vi "Actor Queue.vi"(6 "Creator Queue":refnum<data-value>, 8 "Creator Queue Alias":string, 9 "Self Queue Alias":string, 10 "Queue of Self Queue":refnum<queue>, 11 "Queue":refnum<class "Queue.lvclass">) -> ()   [LabVIEW 2021, in "jettl.lvlib" / "Base Queue.lvlib" / "Base Queue.lvclass"]
uses:
  Base Queue.lvclass
  Queue/Queue.lvclass
  C:/git/jettl/jettl/jettl/jettl/jettl.lvclass
  Msg Strategy/Msg Strategy.lvclass
  C:/git/jettl/jettl/jettl/Queue/Queue.lvclass
  Base Queue.lvclass/Base Queue.ctl
  Self Queue/Self Queue.lvlib
  jettl.lvlib
  Queue Mailbox/Queue Mailbox.lvlib
  Last Ack Created Queue Msg Strategy/Last Ack Created Queue Msg Strategy.lvlib
  Last Ack Creator Queue Msg Strategy/Last Ack Creator Queue Msg Strategy.lvlib
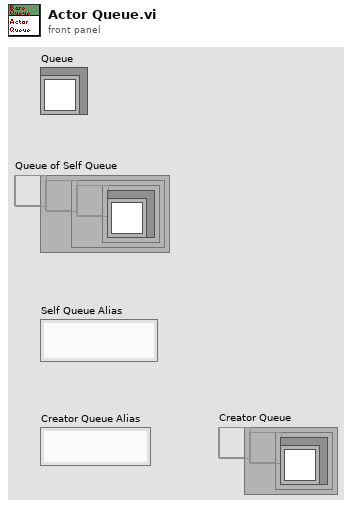
[diagram p1: front panel]
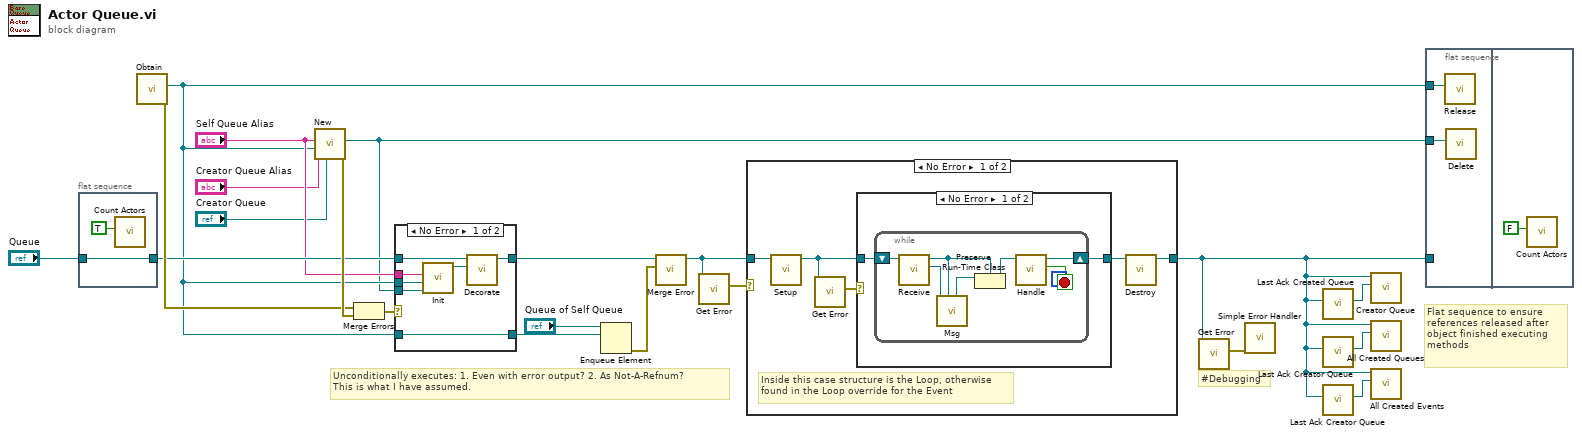
[diagram p0: block diagram]
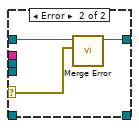
[diagram p2: hidden frame]
diagram:
  # "Flat sequence to ensure references released after object finished executing methods"
  # "#Debugging"
  # "Unconditionally executes: 1. Even with error output? 2. As Not-A-Refnum?\nThis is what I have assumed."
  n1 = flat-sequence {
    tunnel: [w22] -> w11
    tunnel: "Queue" -> [w22]
    frame #0 {
      n2 = call "Count Actors.vi"("Increment?"=TRUE) -> ()  [unwired: 11 in]
    }
  }
  n3 = call "Obtain.vi"() -> ("error out"=w12:errorcluster, "Self Queue"=w8:refnum<data-value>)  [unwired: 10 in]
  n4 = call "New.vi"("Creator Queue"="Creator Queue", "Creator Queue Alias"="Creator Queue Alias", "Self Queue"=w8, "Self Queue Alias"="Self Queue Alias") -> ("error out"=w13:errorcluster, "Queue Mailbox"=w5:refnum<data-value>)  [unwired: 6 in]
  n5 = Merge Errors(w12, w13) -> (w14:errorcluster)
  n6 = case shown="No Error" w14 {
    selector: w14 -> [_ w32]
    tunnel: [w29 w33] -> w19
    tunnel: w11 -> [w30 w31]
    tunnel: w8 -> [w28 _]
    tunnel: [w28 _] -> w18
    tunnel: w5 -> [w26 _]
    tunnel: "Self Queue Alias" -> [w25 _]
    tunnel: w8 -> [w24 _]
    frame No Error {
      n7 = call "Init.vi"("Queue Mailbox"=w26, "Self Queue"=w24, "Self Queue Alias"=w25) -> ("Base Queue out"=w27:refnum<class "Base Queue.lvclass">)  [unwired: 8 in]
      n8 = call-dynamic "Decorate.vi"("Queue"=w27, "Queue in"=w30) -> ("Queue out"=w29:refnum<class "Queue.lvclass">)  [unwired: 9 in]
    }
    frame Error {
      n9 = call-dynamic "Merge Error.vi"("Error"=w32, "Merge Error in"=w31) -> ("Merge Error out"=w33:refnum<class "Queue.lvclass">)  [unwired: 9 in]
    }
  }
  n10 = Enqueue Element(queue="Queue of Self Queue", element=w18) -> (error out=w20:errorcluster)  [unwired: 2 in, 2 out]
  n11 = call-dynamic "Merge Error.vi"("Error"=w20, "Merge Error in"=w19) -> ("Merge Error out"=w21:refnum<class "Queue.lvclass">)  [unwired: 9 in]
  n12 = call-dynamic "Get Error.vi"("jettl in"=w21) -> ("Error"=w17:errorcluster)  [unwired: 10 in]
  n13 = case shown="No Error" w17 {
    tunnel: w21 -> [w35 w49]
    tunnel: [w34 w49] -> w1
    frame No Error {
      # "Inside this case structure is the Loop, otherwise found in the Loop override for the Event"
      n14 = call-dynamic "Setup.vi"("Setup in"=w35) -> ("Setup out"=w37:refnum<class "Queue.lvclass">)  [unwired: 10 in]
      n15 = call-dynamic "Get Error.vi"("jettl in"=w37) -> ("Error"=w38:errorcluster)  [unwired: 10 in]
      n16 = case shown="No Error" w38 {
        tunnel: [w40 w48] -> w36
        tunnel: w37 -> [w39 w48]
        frame No Error {
          n17 = while "Queue Loop" {
            shift-right: [w47] -> w40
            shift-left: w39 -> [w46]
            stop <- w44 stop-if-true
            n18 = call-dynamic "Receive.vi"("Queue in"=w46) -> ("Msg Strategy"=w45:refnum<class "Msg Strategy.lvclass">, "Queue out"=w43:refnum<class "Queue.lvclass">)  [unwired: 9 in]
            n19 = call-dynamic "Msg.vi"("jettl in"=w43, "Msg Strategy in"=w45) -> ("jettl out"=w41:refnum<class "jettl.lvclass">)  [unwired: 9 in]
            n20 = Preserve Run-Time Class(object in=w41, 2:w43) -> (object out=w42:refnum<class "Queue.lvclass">)  [unwired: 1 in, 1 out]
            n21 = call-dynamic "Handle.vi"("jettl in"=w42) -> ("Destroy?"=w44:bool, "jettl out"=w47:refnum<class "Queue.lvclass">)  [unwired: 9 in]
          }
        }
        frame Error {
        }
      }
      n22 = call-dynamic "Destroy.vi"("jettl in"=w36) -> ("jettl out"=w34:refnum<class "Queue.lvclass">)  [unwired: 10 in]
    }
    frame Error {
    }
  }
  n23 = call-dynamic "Get Error.vi"("jettl in"=w1) -> ("Error"=w10:errorcluster)  [unwired: 10 in]
  n24 = call <vilib>:"Simple Error Handler.vi"("error in (no error)"=w10) -> ()  [unwired: 4 in, 5 out]
  n25 = call "Last Ack Created Queue.vi"("Queue"=w1) -> ("Msg Strategy"=w4:refnum<class "Msg Strategy.lvclass">)  [unwired: 10 in]
  n26 = call "Last Ack Creator Queue.vi"("Queue"=w1) -> ("Msg Strategy"=w3:refnum<class "Msg Strategy.lvclass">)  [unwired: 10 in]
  n27 = call "Last Ack Creator Queue.vi"("Queue"=w1) -> ("Msg Strategy"=w2:refnum<class "Msg Strategy.lvclass">)  [unwired: 10 in]
  n28 = call-dynamic "Creator Queue.vi"("Msg Strategy"=w4, "Queue in"=w1) -> ()  [unwired: 9 in, 1 out]
  n29 = call-dynamic "All Created Queues.vi"("Msg Strategy"=w3, "Queue in"=w1) -> ()  [unwired: 9 in, 1 out]
  n30 = call-dynamic "All Created Events.vi"("Msg Strategy"=w2, "Queue in"=w1) -> ()  [unwired: 9 in, 1 out]
  n31 = flat-sequence {
    tunnel: w5 -> [w50]
    tunnel: w8 -> [w51]
    tunnel: w1 -> [_]
    frame #0 {
      n32 = call "Release.vi"("Self Queue"=w51) -> ()  [unwired: 10 in, 1 out]
      n33 = call "Delete.vi"("Queue Mailbox"=w50) -> ()  [unwired: 10 in, 1 out]
    }
    frame #1 {
      n34 = call "Count Actors.vi"("Increment?"=FALSE) -> ()  [unwired: 11 in]
    }
  }
